vi "svx_Orbit and Timebase Segment (Reference).vi"(5 "reset? (F)":bool, 6 "end reach?":bool, 8 "error in (no error)":errorcluster, 9 "indice":cluster{"start":i32, "length":i32}, 11 "order data":dbl[](array[numeric])) -> (0 "error out":errorcluster, 3 "order data out":dbl[](array[numeric]))   [LabVIEW 2017]
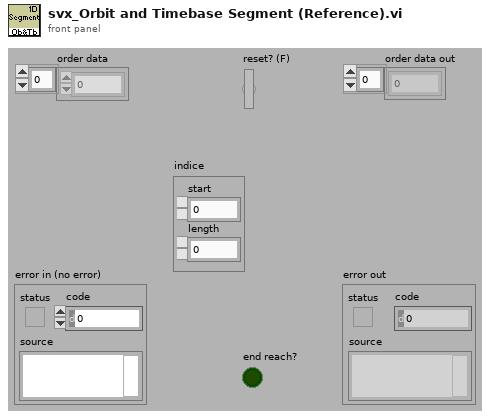
[diagram p1: front panel]
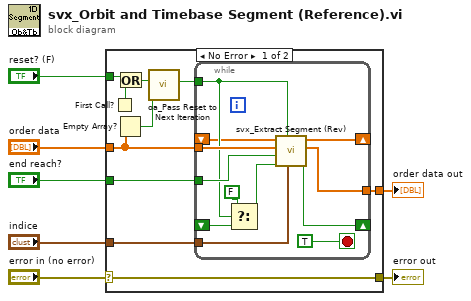
[diagram p0: block diagram]
diagram:
  n1 = case shown="No Error" "error in (no error)" {
    selector: "error in (no error)" -> [w15 w30]
    tunnel: "order data" -> [w14 _]
    tunnel: "reset? (F)" -> [w17 _]
    tunnel: [w15 w30] -> w4
    tunnel: "end reach?" -> [w10 _]
    tunnel: "indice" -> [w9 _]
    tunnel: [w8 _] -> w2
    frame No Error {
      n2 = First Call?() -> (First Call?: T/F=w16:bool)
      n3 = Empty Array?(array=w14) -> (empty?=w12:bool)
      n4 = Or(x=w17, y=w16) -> (x .or. y?=w13:bool)
      n5 = call <vilib>:"oa_Pass Reset to Next Iteration.vi"("trigger"=w12, "reset?(F)"=w13) -> ("reset out"=w11:bool)  [unwired: 9 in]
      n6 = while {
        tunnel: w14 -> [w28]
        shift-right: [w27] -> _
        shift-left: _ -> [w18]
        tunnel: w11 -> [w20]
        shift-right: [w25] -> _
        shift-left: _ -> [w21]
        tunnel: w10 -> [w26]
        tunnel: w9 -> [w24]
        tunnel: [w23] -> w8
        stop <- TRUE stop-if-true
        n7 = Select(t=FALSE, s=w20, f=w21) -> (s? t:f=w22:bool)
        n8 = call <vilib>:"svx_Extract Segment (Rev).vi"("indice"=w24, "reset?"=w20, "old end reached"=w22, "end reached"=w26, "data in"=w28, "old order data"=w18) -> ("end reached out"=w25:bool, "data out"=w23:dbl[], "remaining data"=w27:dbl[])  [unwired: 3 in]
      }
    }
    frame Error {
    }
  }
  "order data out" <- w2
  "error out" <- w4
